vi "adresse + W.vi"(11 "adresse + Write":u8 format="%x") -> (3 "Adresse + command byte":bool[](array[boolean]))   [LabVIEW 2019]
uses:
  <vilib>/rvi/eio/common/nirviEmuTemplateMethod_errors.vi
  <vilib>/eio/EIONode/EIONode.xnode
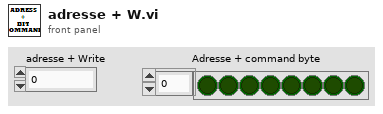
[diagram p1: front panel]
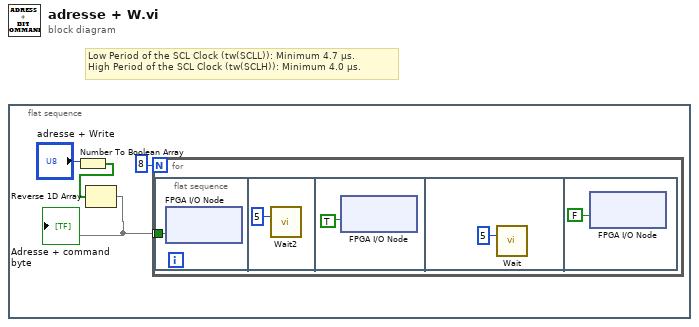
[diagram p0: block diagram]
diagram:
  # "Low Period of the SCL Clock (tw(SCLL)): Minimum 4.7 µs.\nHigh Period of the SCL Clock (tw(SCLH)): Minimum 4.0 µs."
  n1 = flat-sequence {
    frame #0 {
      n2 = Number To Boolean Array(number="adresse + Write") -> (Boolean array=w2:bool[])
      n3 = Reverse 1D Array(array=w2) -> (reversed array=w1:bool[])
      "Adresse + command byte" <- w1
      n4 = for {
        N: 8 -> [_]
        tunnel: w1 -> [w5] mode=indexing
        n5 = flat-sequence {
          tunnel: w5 -> [w6]
          frame #0 {
            n6 = xnode "FPGA I/O Node"("SDA"=w6) -> ()  [unwired: 1 in, 1 out]
          }
          frame #1 {
            n7 = call "Wait2"("Count(uSec)"=u32 5 ("Count(Ticks)")) -> ()  [unwired: 1 out]
          }
          frame #2 {
            n8 = xnode "FPGA I/O Node"("SCL"=TRUE) -> ()  [unwired: 1 in, 1 out]
          }
          frame #3 {
            n9 = call "Wait"("Count(uSec)"=u32 5 ("Count(Ticks)")) -> ()  [unwired: 1 out]
          }
          frame #4 {
            n10 = xnode "FPGA I/O Node"("SCL"=FALSE) -> ()  [unwired: 1 in, 1 out]
          }
        }
      }
    }
  }
